vi "Averaged_Rot_Measure_Main_v1.vi"() -> ()   [LabVIEW 2021]
uses:
  Config_File_Paths.ctl
  ZI_Data.ctl
  <vilib>/Utility/file.llb/Write Delimited Spreadsheet (DBL).vi
  <vilib>/measure/maspectr.llb/FFT Spectrum (Real-Im) for 1 Chan.vi
  <vilib>/Analysis/NI_AALPro.lvlib
  <vilib>/measure/NI_MAPro.lvlib
panel:
  out "averaged spectrum":waveform(dbl)[](graph)
  out "single spectrum":waveform(dbl)[](graph)
  out "single differ":cluster{"Time":dbl[], "X":dbl[]}[](graph)
  out "single abs":cluster{"Time":dbl[], "X":dbl[]}[](graph)
  out "averaged rot":cluster{"Time":dbl[], "X":dbl[]}[](graph)
  out "single rot":cluster{"Time":dbl[], "X":dbl[]}[](graph)
  in  "Resource Address":T1={"ZI Address"="DEV714", "VISA Keithley"="", "VISA Arduino PG"=""}
  in  "error in":errorcluster
  in  "Config files paths":T2={"ZI config file (.ini)"="Config_Ver_1\\Zurich_params.ini", "Keithley config file (.ini)"="Config_Ver_1\\Keithley_params.ini", "Arduino config file (.ini)"="Config_Ver_1\\pulse_sequence.ini"}
  in  "Time unit":string(combo)="ms"
  out "loading":dbl(slide) scale=0.0..100.0
  in  "Number of averages":i32=1
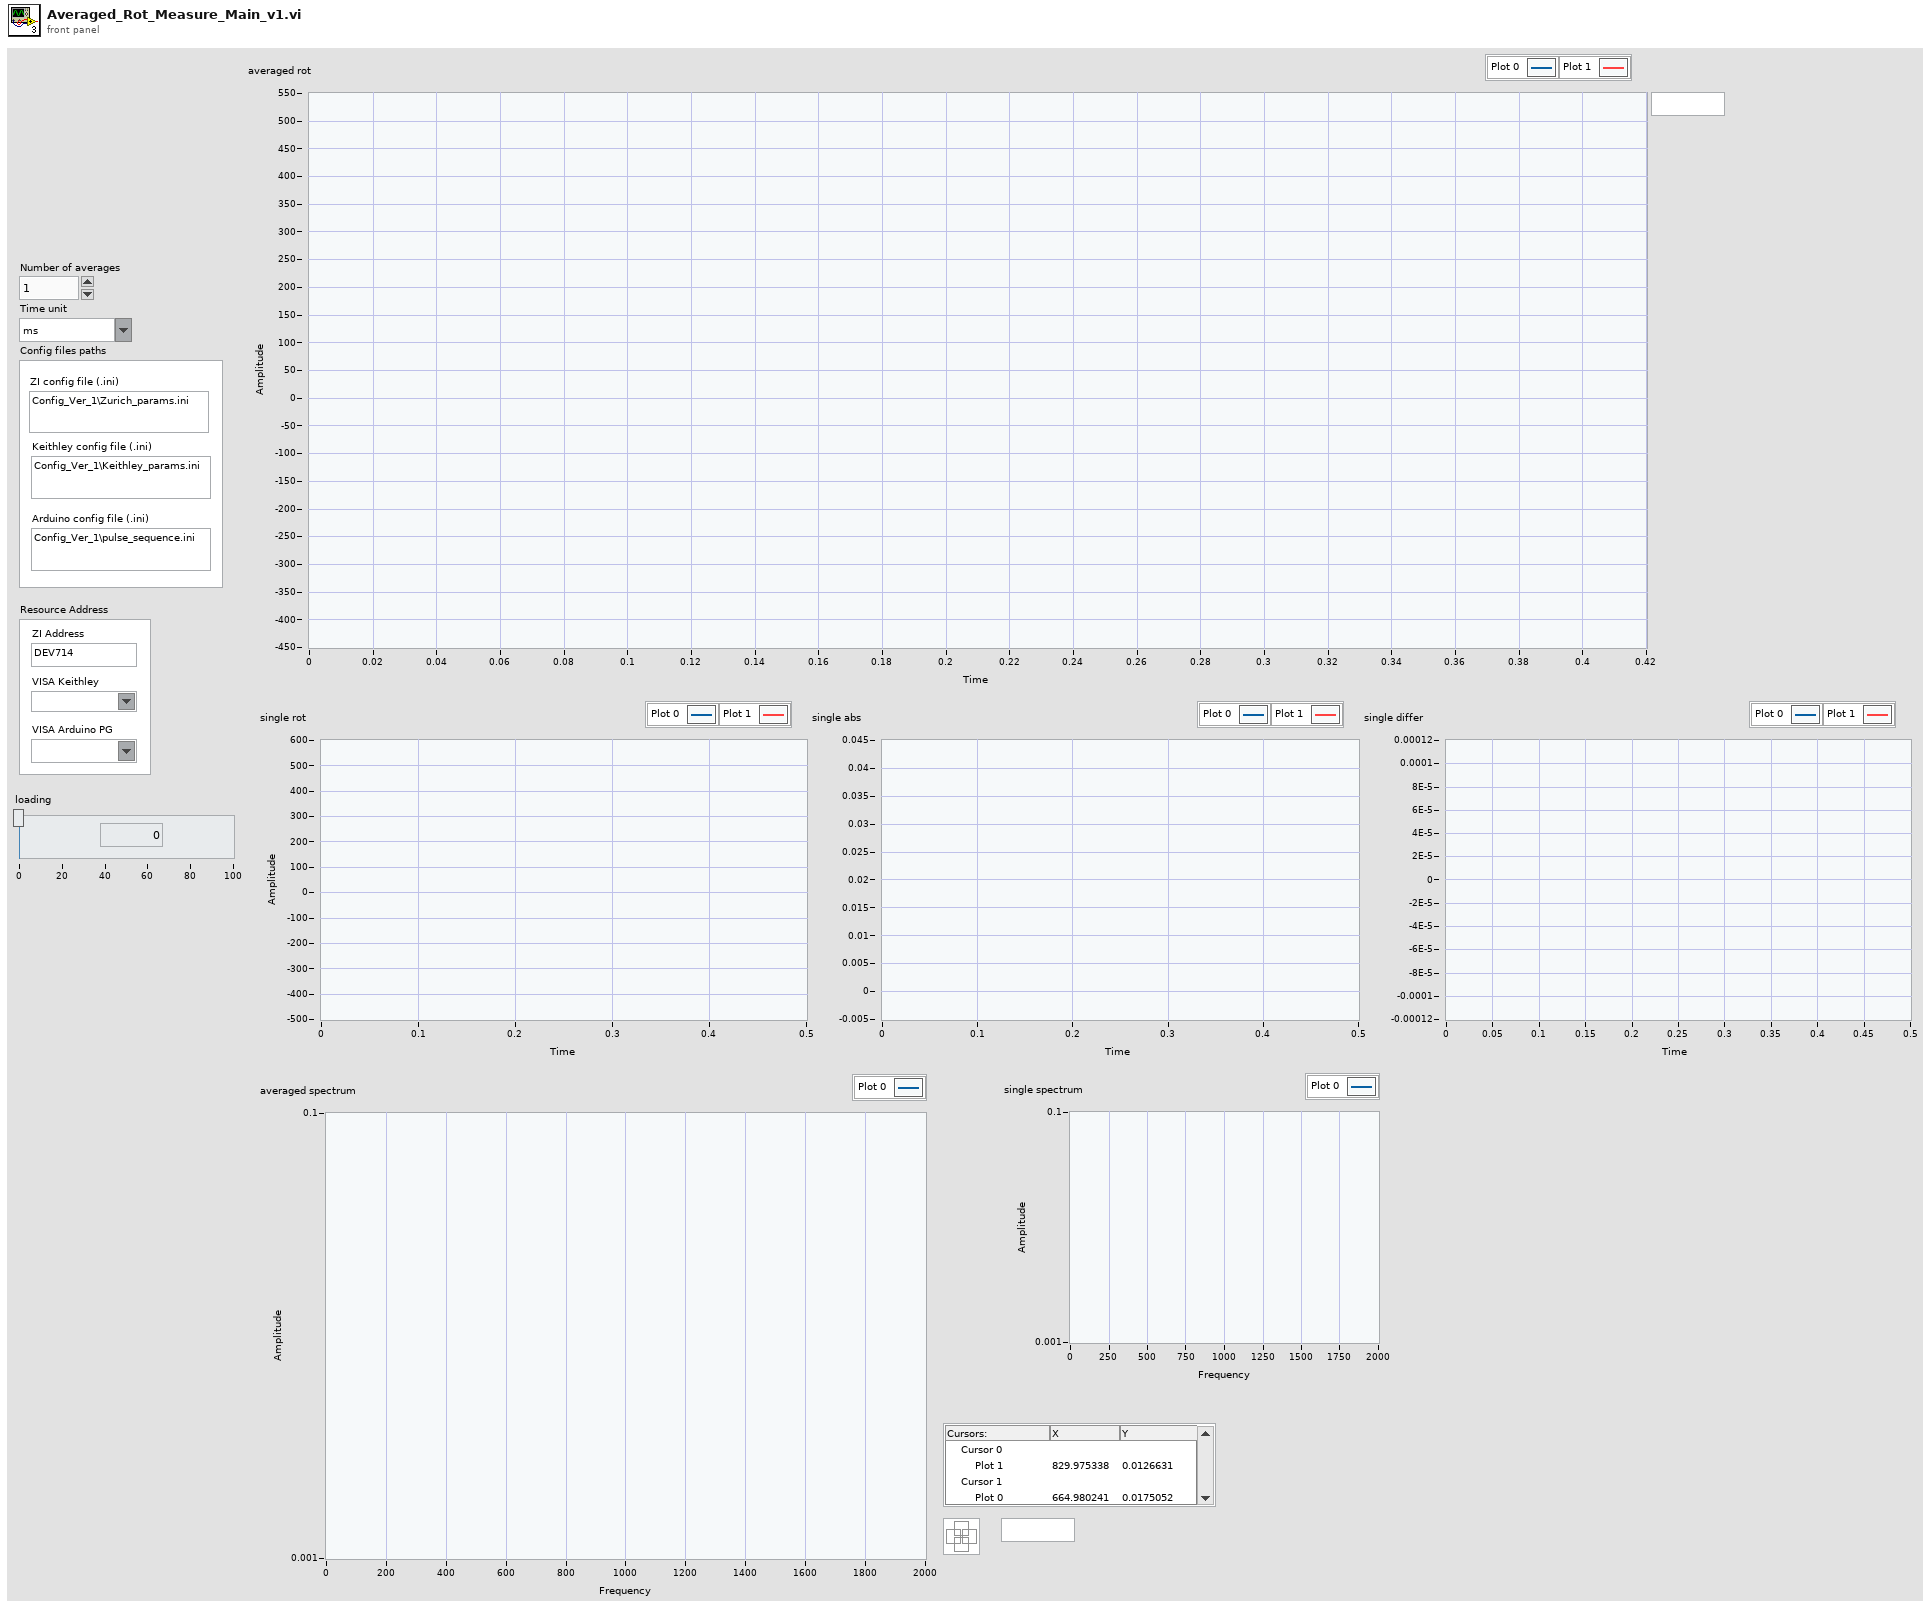
[diagram p1: front panel]
types:
  T1 = cluster{"ZI Address":string, "VISA Keithley":refnum<visa-resource-name>, "VISA Arduino PG":refnum<visa-resource-name>}
  T2 = typedef "Config_File_Paths.ctl" = cluster{"ZI config file (.ini)":string, "Keithley config file (.ini)":string, "Arduino config file (.ini)":string}
  T3 = typedef "ZI_Data.ctl" = cluster{"R":dbl[], "Theta":dbl[], "X":dbl[], "Y":dbl[], "AuxIn0":dbl[], "AuxIn1":dbl[], "Frequency":dbl[], "DIO":dbl[], "Time":dbl[]}
  T4 = typedef "Resources.ctl" = cluster{"ZI Handle":T5, "ZI ModHandle":T6, "VISA arduino":refnum<visa-resource-name>, "VISA Keithley":refnum<visa-resource-name>}
  T5 = typedef "Zurich Instruments LabOne.lvlib/ziTypeHandle.ctl" = cluster{"handleValid":bool, "Conn":u64, "Path Prefix":string, "Handle":u64, "Connected":bool, "Clockbase(s)":dbl}
  T6 = typedef "Zurich Instruments LabOne.lvlib/ziTypeModHandle.ctl" = cluster{"handleValid":bool, "Conn":u64, "ModHandle":u64, "moduleID":string, "Path Prefix":string}
  T7 = typedef "Cutted_Data.ctl" = cluster{"X":dbl[], "Y":dbl[], "Time":dbl[]}
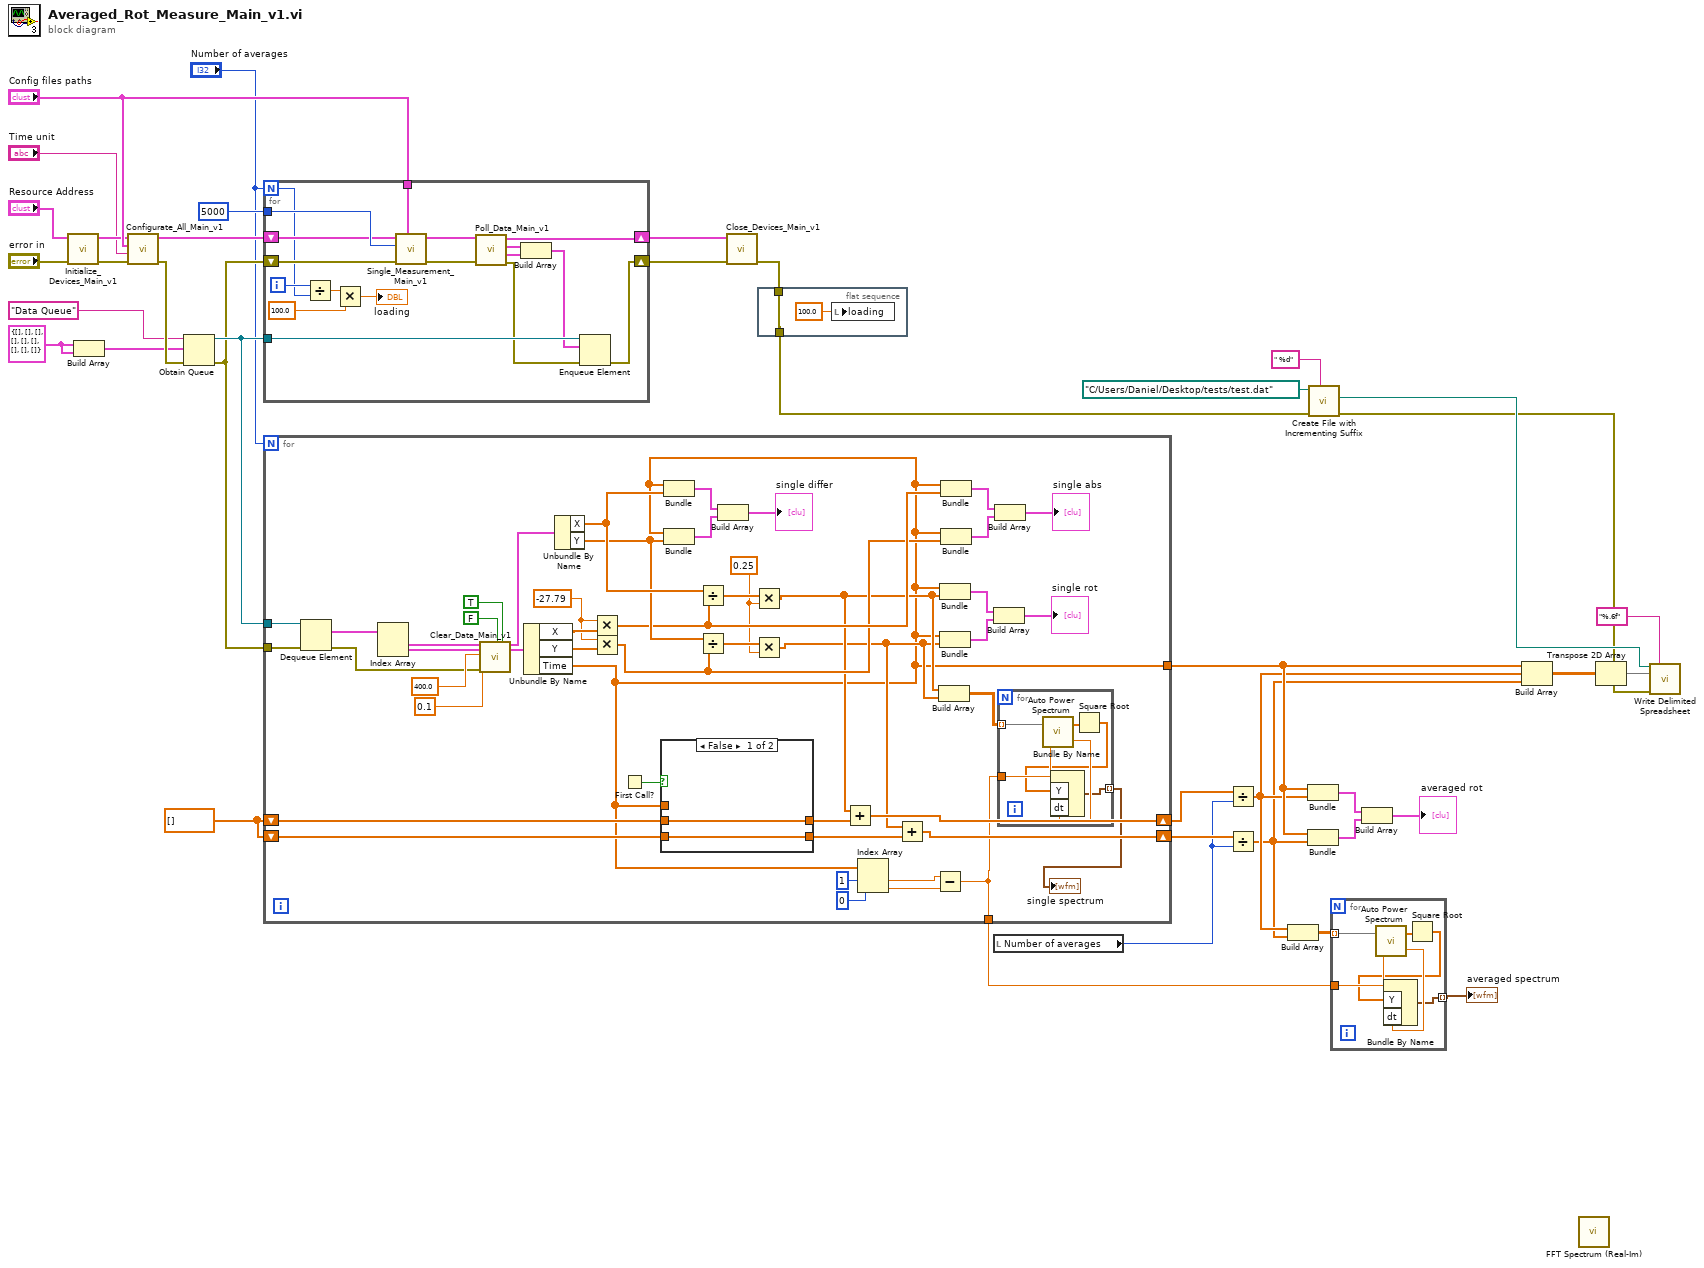
[diagram p0: block diagram]
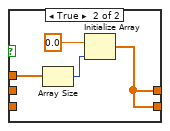
[diagram p2: hidden frame]
diagram:
  w23 = dbl[] []
  w27 = T3 {"R"=[], "Theta"=[], "X"=[], "Y"=[], "AuxIn0"=[], "AuxIn1"=[], "Frequency"=[], "DIO"=[], "Time"=[]} ("ZI Data")
  n1 = call "Initialize_Devices_Main_v1.vi"("error in"="error in", "Resource Address"="Resource Address") -> ("error out"=w31:errorcluster, "Resources"=w32:T4)  [unwired: 8 in]
  n2 = Build Array(w27, w27) -> (w26:T3[])
  n3 = call "Configurate_All_Main_v1.vi"("error in"=w31, "Time unit"="Time unit", "Config files paths"="Config files paths", "Resources in"=w32) -> ("error out"=w29:errorcluster, "Resources out"=w37:T4)  [unwired: 4 in, 2 out]
  n4 = Obtain Queue(name (unnamed)="Data Queue", element data type=w26, error in (no error)=w29) -> (queue out=w25:refnum<queue>, error out=w24:errorcluster)  [unwired: 2 in, 1 out]
  n5 = for {
    N: "Number of averages" -> [w49]
    shift-right: [w51] -> w38
    shift-left: w37 -> [w55]
    shift-right: [w40] -> w39
    shift-left: w24 -> [w54]
    tunnel: "Config files paths" -> [w57]
    tunnel: u64 5000 ("Timeout [ms]") -> [w56]
    tunnel: w25 -> [w45]
    i -> [w50]
    n6 = Divide(x=w50, y=w49) -> (x/y=w48:dbl)
    n7 = Multiply(x=w48, y=100.0) -> (x*y=→"loading":dbl)
    n8 = call "Single_Measurement_Main_v1.vi"("Config files paths"=w57, "error in"=w54, "Timeout [ms]"=w56, "Resources In"=w55) -> ("error out"=w52:errorcluster, "Resources Out"=w53:T4)  [unwired: 6 in]
    n9 = call "Poll_Data_Main_v1.vi"("error in"=w52, "Resources in"=w53) -> ("error out"=w41:errorcluster, "ZI Data 3"=w43:T3, "ZI Data 0"=w44:T3, "Resources out"=w51:T4)  [unwired: 6 in]
    n10 = Build Array(w44, w43) -> (w42:T3[])
    n11 = Enqueue Element(queue=w45, element=w42, error in (no error)=w41) -> (error out=w40:errorcluster)  [unwired: 1 in, 2 out]
  }
  n12 = for {
    N: "Number of averages" -> [_]
    tunnel: w25 -> [w105]
    tunnel: w24 -> [w104]
    shift-right: [w88] -> w20
    shift-left: w23 -> [w92]
    shift-right: [w87] -> w21
    shift-left: w23 -> [w91]
    tunnel: [w64] -> w9
    tunnel: [w58] -> w4
    w68 = 0.25
    w73 = -27.79
    n13 = Dequeue Element(queue=w105, error in (no error)=w104) -> (element=w103:T3[], error out=w98:errorcluster)  [unwired: 1 in, 2 out]
    n14 = Index Array(array=w103) -> (element #1=w102:T3, element #2=w101:T3)  [unwired: 2 in]
    n15 = call "Clear_Data_Main_v1.vi"("ZI Data 0"=w102, "ZI Data 3"=w101, "Time Of Collected Data (ms)"=400.0, "Crosstalk Tolerance"=0.1, "error in"=w98, "Fixed Number Of Points"=FALSE, "Check Phase Mismatch"=TRUE) -> ("Cutted Data"=w95:T7, "Cutted Data 3"=w94:T7)  [unwired: 7 in, 4 out]
    n16 = Unbundle By Name(w94) -> ("X"=w74:dbl[], "Y"=w75:dbl[], "Time"=w64:dbl[])
    n17 = Unbundle By Name(w95) -> ("X"=w77:dbl[], "Y"=w76:dbl[])
    n18 = Multiply(x=w73, y=w74) -> (x*y=w72:dbl[])
    n19 = Multiply(x=w73, y=w75) -> (x*y=w71:dbl[])
    n20 = First Call?() -> (First Call?: T/F=w93:bool)
    n21 = case shown="False" w93 {
      tunnel: w64 -> [_ w117]
      tunnel: w92 -> [w113 _]
      tunnel: [w113 w114] -> w89
      tunnel: [w112 w114] -> w90
      tunnel: w91 -> [w112 _]
      frame False {
      }
      frame True {
        n22 = Array Size(array=w117) -> (size(s)=w115:i32)
        n23 = Initialize Array(0.0 ("element"), w115) -> (w114:dbl[])
      }
    }
    n24 = Bundle("Time"=w64, "X"=w77) -> (w80:cluster{"Time":dbl[], "X":dbl[]})  [unwired: 1 in]
    n25 = Bundle("Time"=w64, "Y"=w76) -> (w79:cluster{"Time":dbl[], "Y":dbl[]})  [unwired: 1 in]
    n26 = Divide(x=w77, y=w72) -> (x/y=w70:dbl[])
    n27 = Divide(x=w76, y=w71) -> (x/y=w69:dbl[])
    n28 = Build Array(w80, w79) -> (→"single differ":cluster{"Time":dbl[], "Y":dbl[]}[])
    n29 = Multiply(x=w70, y=w68) -> (x*y=w67:dbl[])
    n30 = Multiply(x=w69, y=w68) -> (x*y=w66:dbl[])
    n31 = Add(x=w67, y=w89) -> (x+y=w88:dbl[])
    n32 = Index Array(array=w64, index #1=1 ("index"), index #2=0 ("index")) -> (element #1=w61:dbl, element #2=w60:dbl)
    n33 = Add(x=w66, y=w90) -> (x+y=w87:dbl[])
    n34 = Subtract(x=w61, y=w60) -> (x-y=w58:dbl)
    n35 = Build Array(w67, w66) -> (w65:dbl[][])
    n36 = Bundle("Time"=w64, w67) -> (w86:cluster{"Time":dbl[], dbl[]})  [unwired: 1 in]
    n37 = Bundle("Time"=w64, w66) -> (w85:cluster{"Time":dbl[], dbl[]})  [unwired: 1 in]
    n38 = Bundle("Time"=w64, w72) -> (w83:cluster{"Time":dbl[], dbl[]})  [unwired: 1 in]
    n39 = Bundle("Time"=w64, w71) -> (w82:cluster{"Time":dbl[], dbl[]})  [unwired: 1 in]
    n40 = Build Array(w86, w85) -> (→"single rot":cluster{"Time":dbl[], dbl[]}[])
    n41 = Build Array(w83, w82) -> (→"single abs":cluster{"Time":dbl[], dbl[]}[])
    n42 = for {
      tunnel: w65 -> [w111] mode=indexing
      tunnel: w58 -> [w110]
      tunnel: [w108] -> w59 mode=indexing
      n43 = call <vilib>:"Auto Power Spectrum.vi"("dt"=w110, "Signal (V)"=w111) -> ("df"=w109:dbl, "Power Spectrum (V^2 rms)"=w107:dbl[])
      n44 = Square Root(x=w107) -> (sqrt(x)=w106:dbl[])
      n45 = Bundle By Name("Y"=w106, "dt"=w109) -> (w108:waveform(dbl))  [unwired: 1 in]
    }
    "single spectrum" <- w59
  }
  n46 = call "Close_Devices_Main_v1.vi"("error in"=w39, "Resources in"=w38) -> ("error out"=w2:errorcluster)  [unwired: 9 in]
  n47 = flat-sequence {
    tunnel: [w118] -> w1
    tunnel: w2 -> [w118]
    frame #0 {
      n48 = local write "loading"(100.0 ("loading")) -> ()
    }
  }
  n49 = local read "Number of averages"() -> (w19:i32)
  n50 = Divide(x=w20, y=w19) -> (x/y=w7:dbl[])
  n51 = Divide(x=w21, y=w19) -> (x/y=w6:dbl[])
  n52 = Build Array(w7, w6) -> (w5:dbl[][])
  n53 = Bundle("Time"=w9, w7) -> (w16:cluster{"Time":dbl[], dbl[]})  [unwired: 1 in]
  n54 = Bundle("Time"=w9, w6) -> (w17:cluster{"Time":dbl[], dbl[]})  [unwired: 1 in]
  n55 = call <vilib>:"Create File with Incrementing Suffix.vi"("format string (\" (%d)\")"=" %d" ("format string (\" (%d)\")"), "error in (no error)"=w1, "file path"=path "C:/Users/Daniel/Desktop/tests/test.dat") -> ("error out"=w8:errorcluster, "actual path"=w10:path)  [unwired: 6 in, 1 out]
  n56 = for {
    tunnel: w5 -> [w125] mode=indexing
    tunnel: w4 -> [w124]
    tunnel: [w122] -> w3 mode=indexing
    n57 = call <vilib>:"Auto Power Spectrum.vi"("dt"=w124, "Signal (V)"=w125) -> ("df"=w123:dbl, "Power Spectrum (V^2 rms)"=w121:dbl[])
    n58 = Square Root(x=w121) -> (sqrt(x)=w120:dbl[])
    n59 = Bundle By Name("Y"=w120, "dt"=w123) -> (w122:waveform(dbl))  [unwired: 1 in]
  }
  "averaged spectrum" <- w3
  n60 = Build Array(w16, w17) -> (→"averaged rot":cluster{"Time":dbl[], dbl[]}[])
  n61 = Build Array(w9, w7, w6) -> (w13:dbl[][])
  n62 = call-poly <vilib>:"FFT Spectrum (Real-Im).vi"() -> ()  [unwired: 7 in, 5 out]
  n63 = Transpose 2D Array(2D array=w13) -> (transposed array=w12:dbl[][])
  n64 = call-poly <vilib>:"Write Delimited Spreadsheet.vi"("file path (dialog if empty)"=w10, "format (%.3f)"="%.6f", "2D data"=w12, "error in (no error)"=w8) -> ()  [unwired: 10 in, 2 out]
